vi "SHUA.vi"(3 "pass/faill input":string="NG", 4 "索引 (列)":i32=6, 5 "real report":refnum<vi>) -> (1 "PASS&FAIL":string, 2 "引用输出":refnum<vi>)   [LabVIEW 2018]
panel:
  out "子数组":string[](array[string])
  out "数组 3":bool[](array[boolean])
  out "数组 4":u32[](array[colorbox])
  out "输出簇":cluster{"row":i32, "h":i32}
  out "数组 2":bool[](array[boolean])
  out "项名":string[][](array[string])
  out "数组":string[](array[string])
  in  "TEST":i32(listbox)
  in  "real report":i32(listbox)
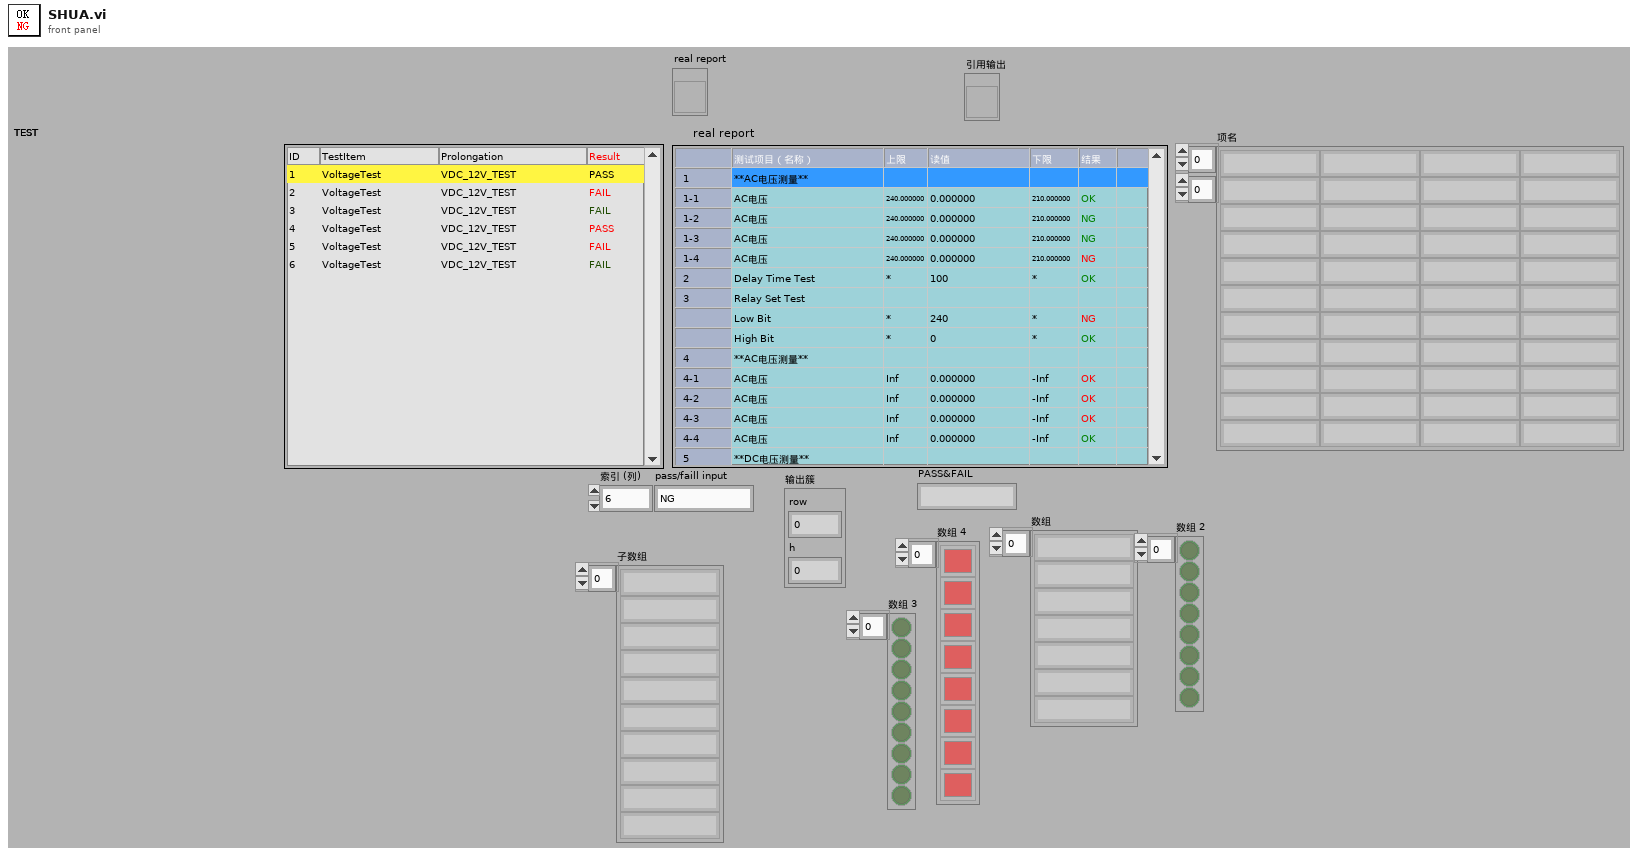
[diagram p1: front panel]
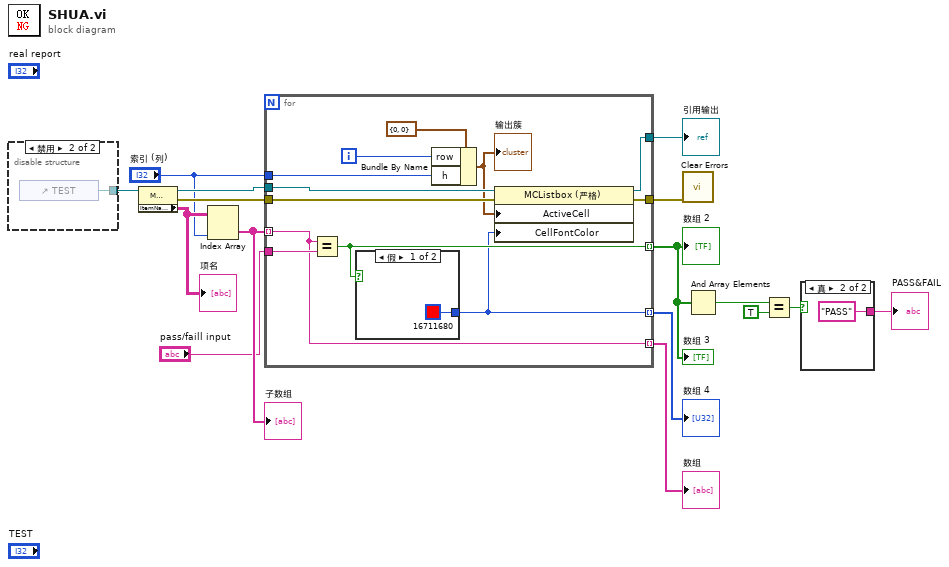
[diagram p0: block diagram]
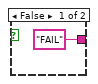
[diagram p2: hidden frame]
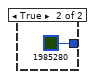
[diagram p3: hidden frame]
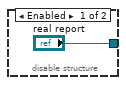
[diagram p4: hidden frame]
diagram:
  n1 = disable-structure shown="禁用" {
    disable-tunnel: ["real report" w18] -> w16
    frame Enabled {
    }
    frame Disabled {
      n2 = control-ref of="TEST"() -> (w18:refnum<vi>)
    }
  }
  n3 = property class="MCListbox (严格)"(reference=w16) -> (reference out=w13:refnum<vi>, error out=w11:errorcluster, "ItemNames"=w12:string[][])  [unwired: 1 in]
  "项名" <- w12
  n4 = Index Array(array=w12, index (col)="索引 (列)") -> (element=w14:string[])  [unwired: 1 in]
  "子数组" <- w14
  n5 = for {
    tunnel: w14 -> [w26] mode=indexing
    tunnel: w13 -> [w24]
    tunnel: [w29] -> w8 mode=indexing
    tunnel: w11 -> [w22]
    tunnel: [w25] -> w1
    tunnel: "索引 (列)" -> [w28]
    tunnel: "pass/faill input" -> [w27]
    tunnel: [w26] -> w4 mode=indexing
    tunnel: [w19] -> w2 mode=indexing
    tunnel: [w23] -> w3
    i -> [w21]
    n6 = Equal?(x=w26, y=w27) -> (x = y?=w29:bool)
    n7 = case shown="假" w29 {
      tunnel: [u32 16711680 u32 1985280] -> w19
      frame False {
      }
      frame True {
      }
    }
    n8 = Bundle By Name(cluster=cluster{"row":i32, "h":i32} {"row"=0, "h"=0} ("输出簇"), "row"=w21, "h"=w28) -> (w20:cluster{"row":i32, "h":i32})
    "输出簇" <- w20
    n9 = property class="MCListbox (严格)"(reference=w24, error in=w22, "ActiveCell"=w20, "CellFontColor"=w19) -> (reference out=w25:refnum<vi>, error out=w23:errorcluster)
  }
  "引用输出" <- w1
  "数组" <- w4
  "数组 2" <- w8
  "数组 4" <- w2
  "数组 3" <- w8
  n10 = call <vilib>:"Clear Errors.vi"("error in (no error)"=w3) -> ()  [unwired: 5 in, 2 out]
  n11 = And Array Elements(Boolean array=w8) -> (logical AND=w7:bool)
  n12 = Equal?(x=w7, y=TRUE) -> (x = y?=w5:bool)
  n13 = case shown="真" w5 {
    tunnel: ["FAIL" "PASS"] -> w15
    frame False {
    }
    frame True {
    }
  }
  "PASS&FAIL" <- w15
